vi "Test-All-JoyStick.vi"() -> ()   [LabVIEW 2023]
doc: "This VI implements the framework and scheduler for your robotics program. It should not be necessary to modify the framework. You are expected to add your code to the VIs called from Robot Main - the ones located in the Team Code folder within the project."
uses:
  <vilib>/Rock Robotics/WPI/DriverStation/WPI_DriverStationRobotMode2.ctl
  Climb/ClimbStates.ctl
  Intake/IntakeStates.ctl
  Robot Global Data.vi
  Wrist/WristGlobal.vi
  Elevator/ElevatorGlobal.vi
  <vilib>/Rock Robotics/WPI/ThirdParty/JAS_Junk/TrajLib/Trajectory_Library.lvlib
panel:
  in  "Tab Control":T1(tab)
  out "Intake Chart":T2(graph)
  out "Intake Top Mot Dmd":dbl format="%9.2f"
  out "Intake Left Mot Dmd":dbl format="%9.1f"
  out "Intake Right Mot Dmd":dbl format="%9.1f"
  out "Intake State":T3
  out "Climb Chart":T2(graph)
  out "Climb Mot Dmd":dbl format="%9.2f"
  out "Climb Angle Deg":dbl format="%9.1f"
  out "Climb At Inner Limit":bool
  out "Climb At Outer Limit":bool
  out "ClimbStates":T4
  out "Wrist Chart":T2(graph)
  out "WristMotorDmd":dbl format="%9.2f"
  out "WristAngle Deg":dbl format="%9.1f"
  out "WristSP Deg":dbl format="%9.1f"
  out "Outer Elevator":T2(graph)
  out "Outer MotorOutDmd":dbl format="%9.2f"
  out "Outer HeightInch":dbl format="%9.1f"
  out "Outer Low Limit Switch":bool
  out "Outer HighLimitSwitch":bool
  out "Outer HeightSP_Inch":dbl format="%9.1f"
  out "Inner Elevator":T2(graph)
  out "Inner MotorOutDmd":dbl format="%9.2f"
  out "Inner HeightInch":dbl format="%9.1f"
  out "Inner Low Limit":bool
  out "Inner HighLimit":bool
  out "Inner HeightSP_Inch":dbl format="%9.1f"
  in  "Intake HaveAlgae":bool
  in  "Intake HaveCoral":bool
  out "Robot Mode":T5
  in  "Finish":bool
  # "Sensor Simulation"
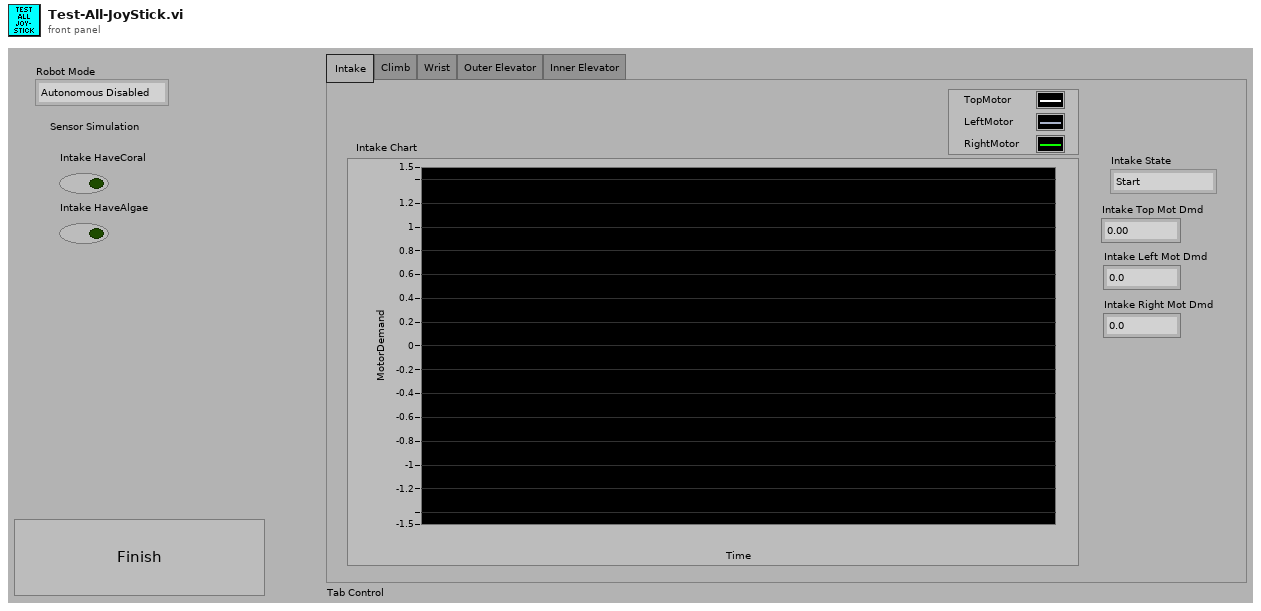
[diagram p1: front panel]
types:
  T1 = enum32{"Intake ", "Climb", "Wrist", "Outer Elevator", "Inner Elevator"}
  T2 = cluster{"ElevatorPosDemandHeight":dbl, "ElevHeightInch":dbl, "MotorDemand":dbl}
  T3 = typedef "IntakeStates.ctl" = enum16{"Start", "WaitForCommand", "IntakeCoral", "IntakeAlgae", "WaitForCoral", "WaitForAlgae", "DepositCoral", "DepositAlgae", "DepositCoralTimer", "DepositAlgaeTimer"}
  T4 = typedef "ClimbStates.ctl" = enum16{"Start", "WaitForCommands", "ClimbRest", "ClimbReach", "ClimbPull"}
  T5 = typedef "WPI_DriverStationRobotMode2.ctl" = enum16{"Autonomous Disabled", "Autonomous Enabled", "Teleop Disabled", "Teleop Enabled", "Disconnected", "Finish", "Test Disabled", "Test Enabled", "Emergency Stopped"}
  T6 = cluster{"MotorDemandTop":dbl, "MotorDemandLeft":dbl, "MotorDemandRight":dbl}
  T7 = cluster{"WristSP Deg 2":dbl, "ClimbPositionDegrees":dbl, "MotorDemand":dbl}
  T8 = cluster{"ElevatorStage3PosDemandHeight":dbl, "Inner  HeightInches":dbl, "Stage3MotorDemand":dbl}
  T9 = cluster{"ElevatorOuterPosDemandHeight":dbl, "Outer ElevHeightInch":dbl, "OuterMotorDemand":dbl}
  T10 = cluster{"CurrentWristSetpoint":dbl, "WritstPositionDegrees":dbl, "MotorDmd":dbl}
  T11 = typedef "WPI_DriverStationMatch Info.ctl" = cluster{"Autonomous Elapsed Seconds":dbl, "TeleOp Elapsed Seconds":dbl, "Disabled Elapsed Seconds":dbl, "Visited Autonomous":bool, "Visited TeleOp":bool, "Visited Disabled":bool, "Autonomous Settings":cluster{"Autonomous Style":enum16{"Iterative", "Independent"}, "VI Refnum":refnum<vi>}}
  T12 = typedef "WPI_DriverStationDerivedRobotMode.ctl" = enum16{"Init", "Execute", "Stop"}
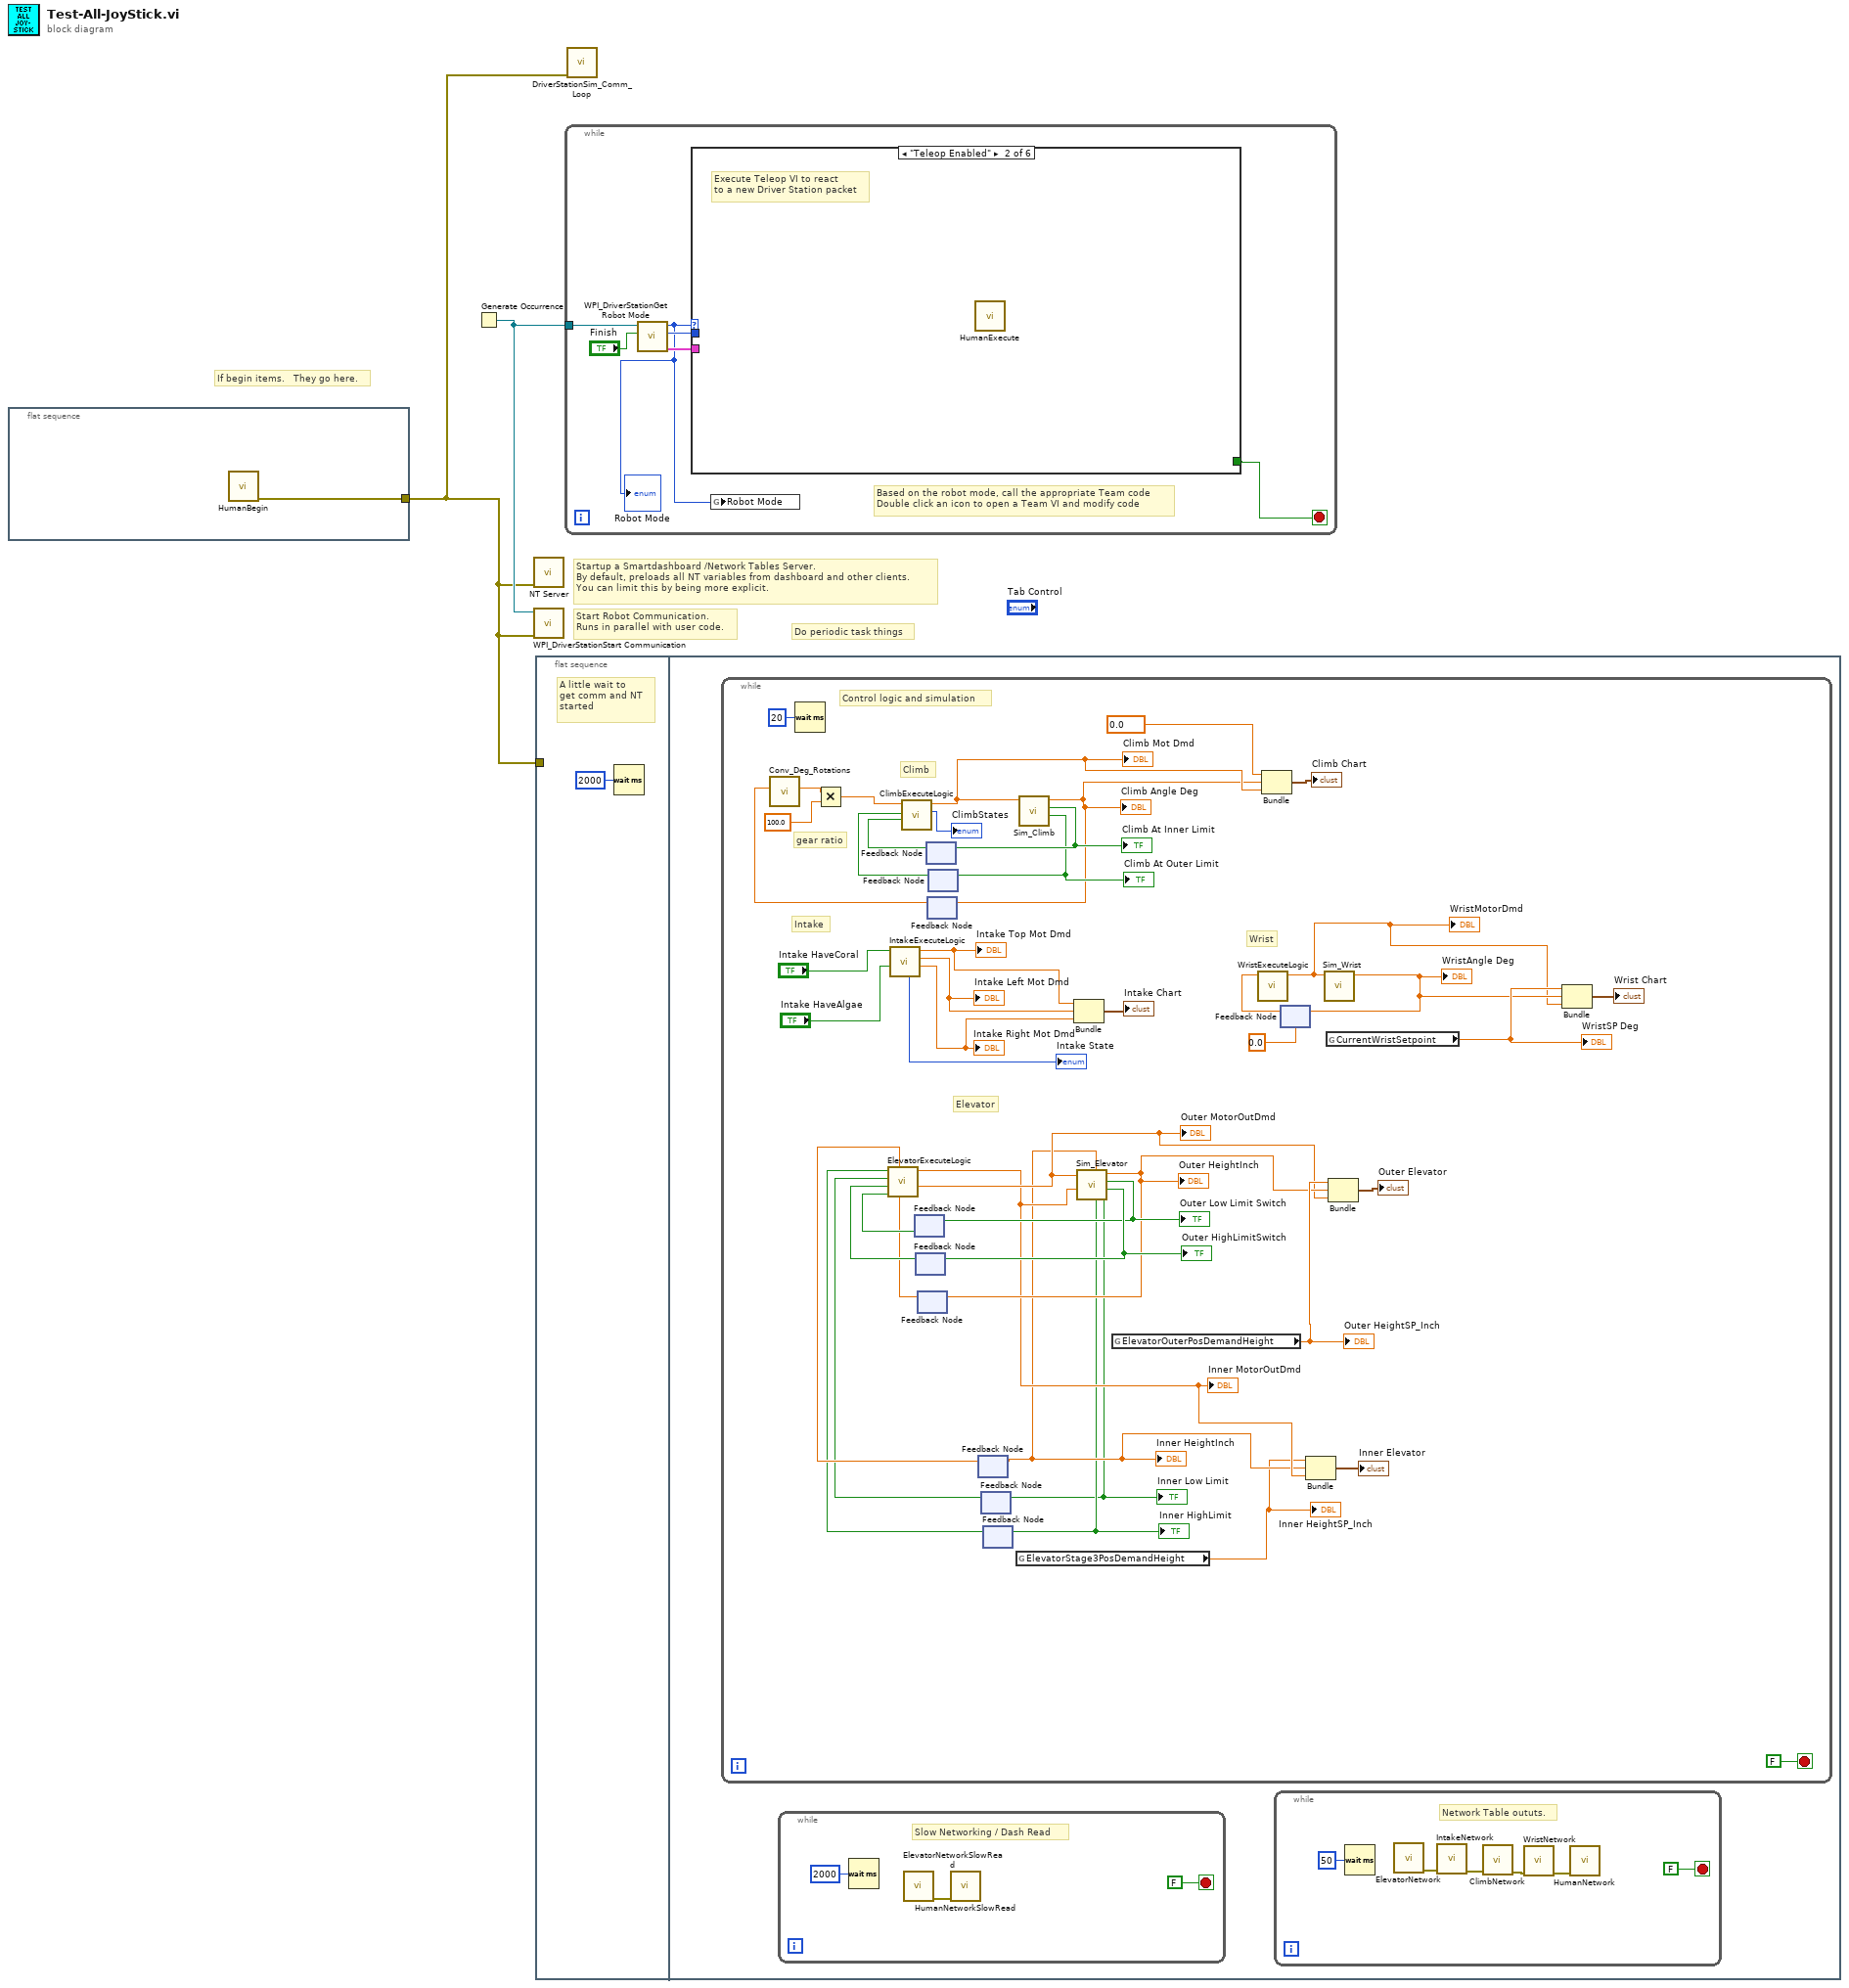
[diagram p0: block diagram]
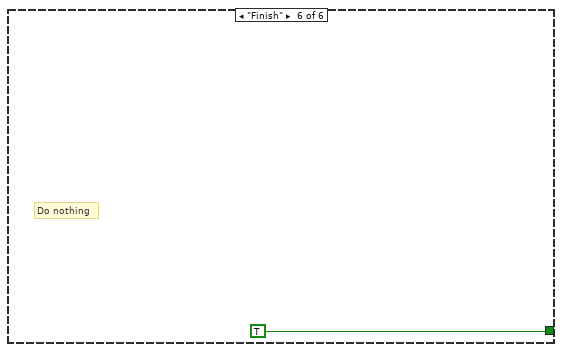
[diagram p6: hidden frame]
diagram:
  # "If begin items.   They go here."
  # "Do periodic task things"
  # "Startup a Smartdashboard /Network Tables Server.\nBy default, preloads all NT variables from dashboard and other clients.\nYou can limit this by being more explicit."
  # "Start Robot Communication.\nRuns in parallel with user code."
  n1 = flat-sequence {
    tunnel: [w3] -> w1
    frame #0 {
      n2 = call "HumanBegin.vi"() -> ("error out"=w3:errorcluster)  [unwired: 11 in]
    }
  }
  n3 = Generate Occurrence() -> (w2:refnum<k4>)
  n4 = call <vilib>:"NT Server.vi"("error in (no error)"=w1) -> ()  [unwired: 10 in, 1 out]
  n5 = call <vilib>:"WPI_DriverStationStart Communication.vi"("error in (no error)"=w1, "occurrence"=w2) -> ()  [unwired: 1 in, 9 out]
  n6 = flat-sequence {
    tunnel: w1 -> [_]
    frame #0 {
      # "A little wait to\nget comm and NT\nstarted"
      n7 = Wait (ms)(milliseconds to wait=u32 2000) -> ()  [unwired: 1 out]
    }
    frame #1 {
      n8 = while {
        stop <- FALSE stop-if-true
        # "Elevator"
        # "Wrist"
        # "Intake"
        # "gear ratio"
        # "Climb"
        # "Control logic and simulation"
        n9 = Wait (ms)(milliseconds to wait=u32 20) -> ()  [unwired: 1 out]
        n10 = call "IntakeExecuteLogic.vi"("HaveAlgaeSensor"="Intake HaveAlgae", "HaveCoralSensor"="Intake HaveCoral") -> ("MotorDemandRight"=w40:dbl, "MotorDemandLeft"=w41:dbl, "MotorDemandTop"=w42:dbl, "CurrentState"=→"Intake State":T3)  [unwired: 6 in]
        "Intake Top Mot Dmd" <- w42
        "Intake Left Mot Dmd" <- w41
        "Intake Right Mot Dmd" <- w40
        n11 = feedback #1() -> (w26:bool)  [unwired: 1 in]
        n12 = feedback #2() -> (w25:bool)  [unwired: 1 in]
        n13 = feedback #3() -> (w24:dbl)  [unwired: 1 in]
        n14 = feedback #4() -> (w48:bool)  [unwired: 1 in]
        n15 = feedback #5() -> (w49:dbl)  [unwired: 1 in]
        n16 = call <vilib>:"Conv_Deg_Rotations.vi"("Degrees"=w49) -> ("Rotations"=w52:dbl)  [unwired: 10 in]
        n17 = Multiply(x=w52, y=100.0) -> (x*y=w45:dbl)
        n18 = feedback #6() -> (w47:bool)  [unwired: 1 in]
        n19 = call "ClimbExecuteLogic.vi"("PullLS"=w48, "ReachLS"=w47, "SensorPosition"=w45) -> ("ClimbStates"=→"ClimbStates":T4, "MotorDemand"=w55:dbl)  [unwired: 6 in, 1 out]
        "Climb Mot Dmd" <- w55
        n20 = feedback #7() -> (w22:dbl)  [unwired: 1 in]
        n21 = feedback #8() -> (w14:bool)  [unwired: 1 in]
        n22 = feedback #9() -> (w16:bool)  [unwired: 1 in]
        n23 = call "ElevatorExecuteLogic.vi"("OuterPositionHeight"=w24, "InnerPositionHeight"=w22, "OuterLowLimitSwitch"=w26, "OuterHighLimitSwitch"=w25, "Stage3LowLimitSwitch"=w14, "Stage3HighLimitSwitch"=w16) -> ("OuterMotorDemand"=w23:dbl, "Stage3MotorDemand"=w21:dbl)  [unwired: 4 in]
        "Outer MotorOutDmd" <- w23
        "Inner MotorOutDmd" <- w21
        n24 = global read "ElevatorGlobal.vi" "ElevatorStage3PosDemandHeight"() -> (w19:dbl)
        "Inner HeightSP_Inch" <- w19
        n25 = call "Sim_Climb.vi"("Motor1 Dmd"=w55) -> ("At Outer Limit"=w53:bool, "At Climbed Limit"=w54:bool, "ClimbPositionDegrees"=w50:dbl)  [unwired: 6 in, 2 out]
        "Climb Angle Deg" <- w50
        "Climb At Inner Limit" <- w54
        "Climb At Outer Limit" <- w53
        n26 = feedback-in #4(w54) -> ()
        n27 = feedback-in #5(w50) -> ()
        n28 = feedback-in #6(w53) -> ()
        n29 = Bundle("MotorDemandTop"=w42, "MotorDemandLeft"=w41, "MotorDemandRight"=w40) -> (→"Intake Chart":T6)  [unwired: 1 in]
        n30 = call "Sim_Elevator.vi"("Inner Demand"=w21, "Outer Dmd"=w23) -> ("Inner At Low Limit"=w15:bool, "HighLimitSwitch"=w31:bool, "Low Limit Switch"=w30:bool, "Outer ElevHeightInch"=w28:dbl, "Inner At High Limit"=w17:bool, "Inner  HeightInches"=w20:dbl)  [unwired: 1 in, 3 out]
        "Outer HeightInch" <- w28
        "Outer Low Limit Switch" <- w30
        "Outer HighLimitSwitch" <- w31
        "Inner HeightInch" <- w20
        "Inner Low Limit" <- w15
        "Inner HighLimit" <- w17
        n31 = feedback-in #1(w30) -> ()
        n32 = feedback-in #2(w31) -> ()
        n33 = feedback-in #3(w28) -> ()
        n34 = feedback-in #7(w20) -> ()
        n35 = feedback-in #8(w15) -> ()
        n36 = feedback-in #9(w17) -> ()
        n37 = global read "ElevatorGlobal.vi" "ElevatorOuterPosDemandHeight"() -> (w29:dbl)
        "Outer HeightSP_Inch" <- w29
        n38 = Bundle("WristSP Deg 2"=0.0, "ClimbPositionDegrees"=w50, "MotorDemand"=w55) -> (→"Climb Chart":T7)  [unwired: 1 in]
        n39 = feedback #10(0.0 ("WritstPositionDegrees")) -> (w36:dbl)
        n40 = call "WristExecuteLogic.vi"("EncoderPos (deg)"=w36) -> ("MotorDmd"=w32:dbl)  [unwired: 9 in, 1 out]
        "WristMotorDmd" <- w32
        n41 = Bundle("ElevatorStage3PosDemandHeight"=w19, "Inner  HeightInches"=w20, "Stage3MotorDemand"=w21) -> (→"Inner Elevator":T8)  [unwired: 1 in]
        n42 = call "Sim_Wrist.vi"("Motor1 Dmd"=w32) -> ("WritstPositionDegrees"=w34:dbl)  [unwired: 6 in, 4 out]
        "WristAngle Deg" <- w34
        n43 = feedback-in #10(w34) -> ()
        n44 = global read "WristGlobal.vi" "CurrentWristSetpoint"() -> (w35:dbl)
        "WristSP Deg" <- w35
        n45 = Bundle("ElevatorOuterPosDemandHeight"=w29, "Outer ElevHeightInch"=w28, "OuterMotorDemand"=w23) -> (→"Outer Elevator":T9)  [unwired: 1 in]
        n46 = Bundle("CurrentWristSetpoint"=w35, "WritstPositionDegrees"=w34, "MotorDmd"=w32) -> (→"Wrist Chart":T10)  [unwired: 1 in]
      }
      n47 = while {
        stop <- FALSE stop-if-true
        # "Slow Networking / Dash Read"
        n48 = Wait (ms)(milliseconds to wait=u32 2000) -> ()  [unwired: 1 out]
        n49 = call "ElevatorNetworkSlowRead.vi"() -> ("error out"=w5:errorcluster)  [unwired: 11 in]
        n50 = call "HumanNetworkSlowRead.vi"("error in (no error)"=w5) -> ()  [unwired: 10 in, 1 out]
      }
      n51 = while {
        stop <- FALSE stop-if-true
        # "Network Table oututs."
        n52 = Wait (ms)(milliseconds to wait=u32 50) -> ()  [unwired: 1 out]
        n53 = call "ElevatorNetwork.vi"() -> ("error out"=w11:errorcluster)  [unwired: 11 in]
        n54 = call "IntakeNetwork.vi"("error in (no error)"=w11) -> ("error out"=w10:errorcluster)  [unwired: 10 in]
        n55 = call "ClimbNetwork.vi"("error in (no error)"=w10) -> ("error out"=w9:errorcluster)  [unwired: 10 in]
        n56 = call "WristNetwork.vi"("error in (no error)"=w9) -> ("error out"=w8:errorcluster)  [unwired: 10 in]
        n57 = call "HumanNetwork.vi"("error in (no error)"=w8) -> ()  [unwired: 10 in, 1 out]
      }
    }
  }
  n58 = while {
    tunnel: w2 -> [w65]
    stop <- w60 stop-if-true
    # "Based on the robot mode, call the appropriate Team code\nDouble click an icon to open a Team VI and modify code"
    n59 = call <vilib>:"WPI_DriverStationGet Robot Mode.vi"("Finish"="Finish", "DS Occurrence"=w65) -> ("Match Info out"=w62:T11, "Call Context"=w64:T12, "Robot Mode"=w61:T5)  [unwired: 7 out]
    "Robot Mode" <- w61
    n60 = case shown="\"Teleop Enabled\"" w61 {
      tunnel: w64 -> [_ _ _ _ _ _]
      tunnel: w62 -> [_ _ _ _ _ _]
      tunnel: [_ _ _ _ _ TRUE] -> w60
      frame "Autonomous Enabled" {
        # "Do nothing...."
      }
      frame "Teleop Enabled" {
        # "Execute Teleop VI to react\nto a new Driver Station packet"
        n61 = call "HumanExecute.vi"() -> ()  [unwired: 11 in, 1 out]
      }
      frame "Test Disabled", "Test Enabled" {
        # "Do nothing"
      }
      frame "Autonomous Disabled", "Teleop Disabled" {
        # "Do nothing."
      }
      frame "Disconnected", Default {
        # "Driver Station packet didn't arrive.\nPossibly useful for diagnostics"
      }
      frame "Finish" {
        # "Do nothing"
      }
    }
    n62 = global write "Robot Global Data.vi" "Robot Mode"(w61) -> ()
  }
  n63 = call <vilib>:"DriverStationSim_Comm_Loop.vi"("error in (no error)"=w1) -> ()  [unwired: 11 in]
